vi "Rec_config magnet move program.vi"(7 "磁铁最低位置":dbl, 8 "error in (no error)":errorcluster caption="错误输入（无错误）", 9 "参数设置 in":T3={"测量模式"=enum."force clamp", "测量起点"=0.0, "数据存放路径"=path "", "加载率(pN/s)"=0.01, "初始转数"=0.0, "最终转数"=0.0, "旋转速度"=0.0, "步长"=0.0, "FC停留时间"=0.0, "实验名称"="", "往返？"=FALSE, "驰豫时间（s）"=0.0, "单位"=enum."分", "测量周期"=0, "驰豫位置"=0.0, "FR每步时间(s)"=0.5, "测量终点"=[], "阶段终点"=[1.4, 1.0, 0.7], "阶段等待时间(s)"=[3.0, 2.0, 1.0], "顶端驰豫时间"=0, "顶端驰豫"=FALSE} {"FR每步时间(s)" min=0.5; "加载率(pN/s)" min=0.01}, 10 "数据存放路径":path, 11 "motor control":T2={"Position no."=1, "Rotaion no."=2, "piezo no."=3, "mg position"=0.0, "mg rotation"=0.0, "piezo position"=0.0, "pos axes"=[], "rot axes"=[], "piezo axes"=[]}) -> (0 "error out":errorcluster caption="错误输出", 2 "mag ctl":T1 {"磁铁运动参数"."FR每步时间(s)" min=0.5; "磁铁运动参数"."加载率(pN/s)" min=0.01})   [LabVIEW 2017]
doc: "该模板用于创建子VI。"
uses:
  device control/device index.ctl
  parameter set for record.ctl
  control/record mode.ctl
  device control/magnet control.ctl
panel:
  # "force ramp"
  # "force ramp"
  # "通用"
  # "force ramp"
  # "force clamp"
  # "磁铁旋转"
  # "force ramp"
  # "force ramp"
  # "通用"
  # "force ramp"
  # "force clamp"
  # "磁铁旋转"
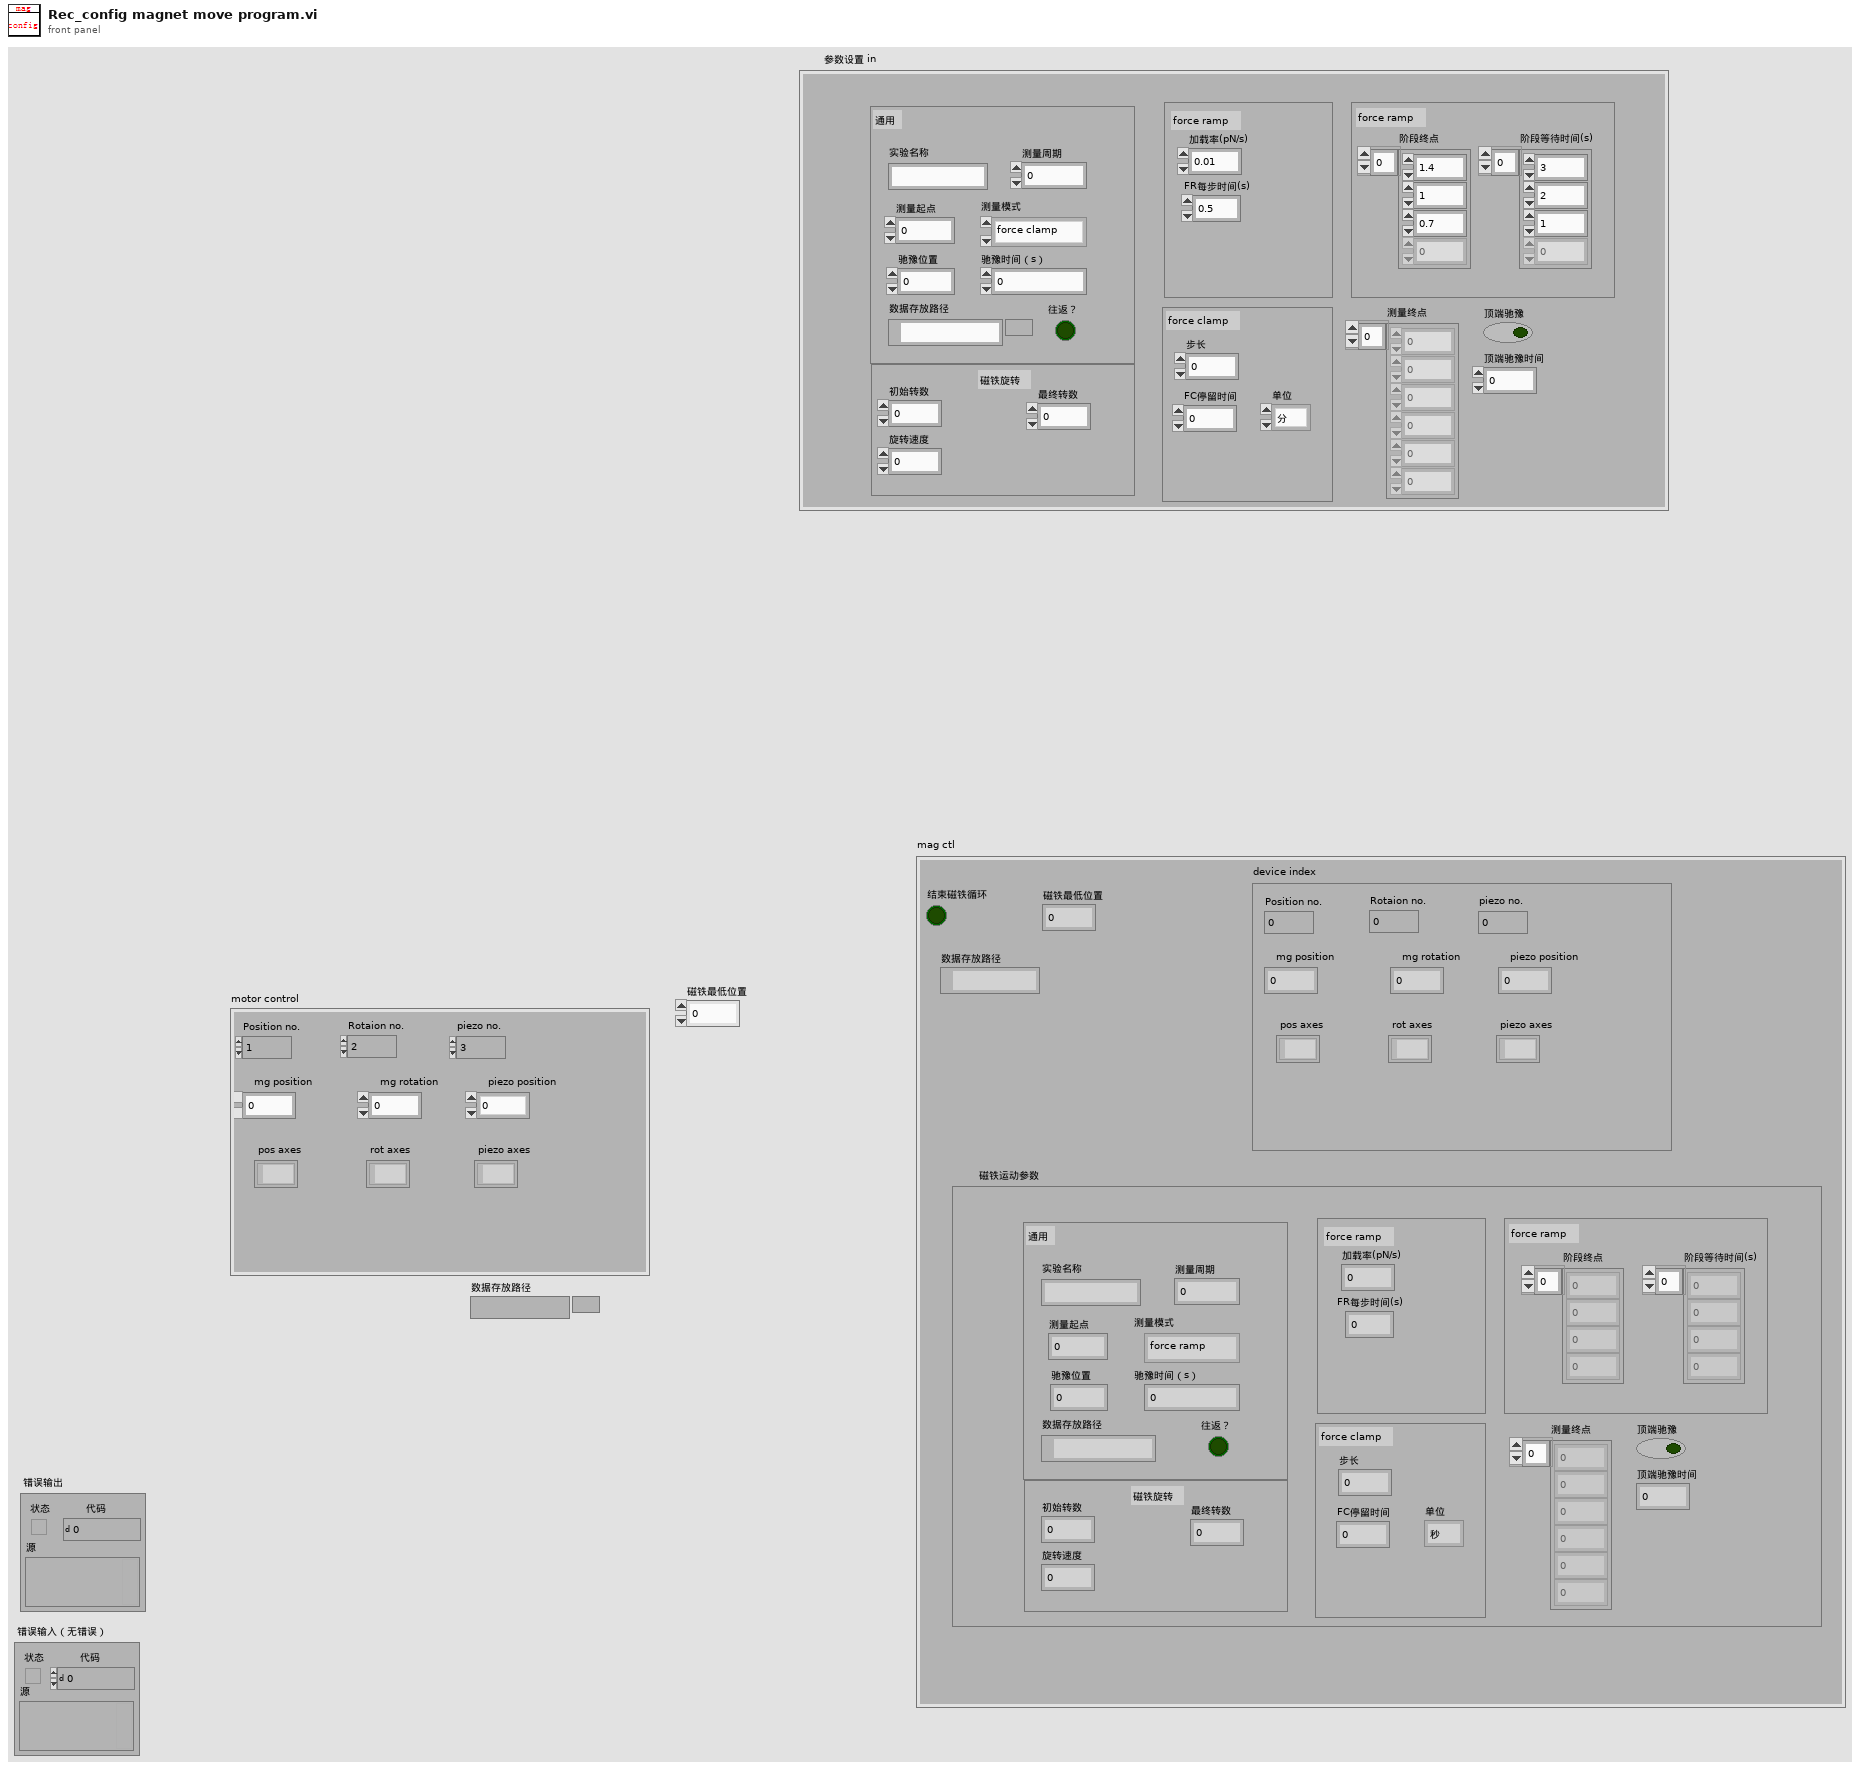
[diagram p1: front panel]
types:
  T1 = typedef "magnet control.ctl" = cluster{"device index":T2, "结束磁铁循环":bool, "磁铁最低位置":dbl, "数据存放路径":path, "磁铁运动参数":T3}
  T2 = typedef "device index.ctl" = cluster{"Position no.":i32, "Rotaion no.":i32, "piezo no.":i32, "mg position":dbl, "mg rotation":dbl, "piezo position":dbl, "pos axes":string[], "rot axes":string[], "piezo axes":string[]}
  T3 = typedef "parameter set for record.ctl" = cluster{"测量模式":T4, "测量起点":dbl, "数据存放路径":path, "加载率(pN/s)":dbl, "初始转数":dbl, "最终转数":dbl, "旋转速度":dbl, "步长":dbl, "FC停留时间":dbl, "实验名称":string, "往返？":bool, "驰豫时间（s）":dbl, "单位":enum16{"秒", "毫秒", "分"}, "测量周期":i32, "驰豫位置":dbl, "FR每步时间(s)":dbl, "测量终点":dbl[], "阶段终点":dbl[], "阶段等待时间(s)":dbl[], "顶端驰豫时间":u32, "顶端驰豫":bool}
  T4 = typedef "record mode.ctl" = enum16{"force ramp", "force clamp", "user-defined", "force-mixed"}
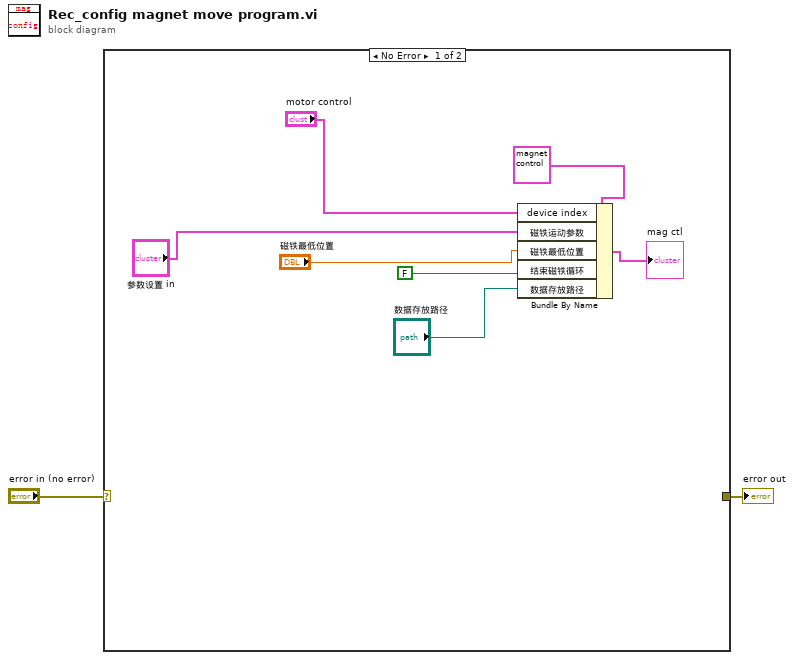
[diagram p0: block diagram]
diagram:
  n1 = case shown="No Error" "error in (no error)" {
    selector: "error in (no error)" -> [_ w10]
    tunnel: [_ w10] -> w1
    frame No Error {
      n2 = Bundle By Name(cluster=T1 {"device index"={"Position no."=0, "Rotaion no."=0, "piezo no."=0, "mg position"=0.0, "mg rotation"=0.0, "piezo position"=0.0, "pos axes"=[], "rot axes"=[], "piezo axes"=[]}, "结束磁铁循环"=FALSE, "磁铁最低位置"=0.0, "数据存放路径"=path "", "磁铁运动参数"={"测量模式"=enum."force ramp", "测量起点"=0.0, "数据存放路径"=path "", "加载率(pN/s)"=0.0, "初始转数"=0.0, "最终转数"=0.0, "旋转速度"=0.0, "步长"=0.0, "FC停留时间"=0.0, "实验名称"="", "往返？"=FALSE, "驰豫时间（s）"=0.0, "单位"=enum."秒", "测量周期"=0, "驰豫位置"=0.0, "FR每步时间(s)"=0.0, "测量终点"=[], "阶段终点"=[], "阶段等待时间(s)"=[], "顶端驰豫时间"=0, "顶端驰豫"=FALSE}} ("mag ctl"), "device index"="motor control", "磁铁运动参数"="参数设置 in", "磁铁最低位置"="磁铁最低位置", "结束磁铁循环"=FALSE, "数据存放路径"="数据存放路径") -> (→"mag ctl":T1)
    }
    frame Error {
    }
  }
  "error out" <- w1
